vi "Constructor.vi"(8 "error in (no error)":errorcluster, 11 "MallardDuck in":refnum<class "MallardDuck.lvclass">) -> (0 "error out":errorcluster, 3 "MallardDuck out":refnum<class "MallardDuck.lvclass">)   [LabVIEW 2013, in "MallardDuck.lvclass"]
uses:
  MallardDuck.lvclass
  FlyWithWings/FlyWithWings.lvclass
  Quack/Quack.lvclass
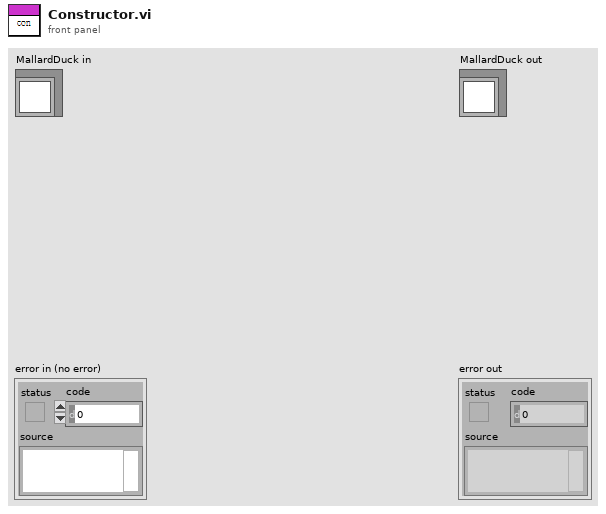
[diagram p1: front panel]
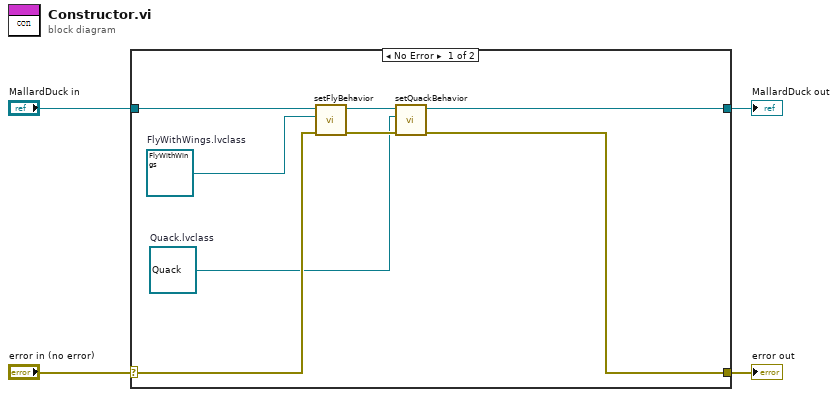
[diagram p0: block diagram]
diagram:
  n1 = case shown="No Error" "error in (no error)" {
    selector: "error in (no error)" -> [w8 w14]
    tunnel: [w7 w14] -> w3
    tunnel: [w10 w13] -> w1
    tunnel: "MallardDuck in" -> [w11 w13]
    frame No Error {
      w5 = refnum<class "Quack.lvclass"> refnum  # Quack.lvclass
      w6 = refnum<class "FlyWithWings.lvclass"> refnum  # FlyWithWings.lvclass
      n2 = call-dynamic "setFlyBehavior.vi"("error in (no error)"=w8, "FlyBehavior.lvclass"=w6, "Duck in"=w11) -> ("error out"=w9:errorcluster, "Duck out"=w12:refnum<class "MallardDuck.lvclass">)  [unwired: 7 in]
      n3 = call-dynamic "setQuackBehavior.vi"("error in (no error)"=w9, "QuackBehavior.lvclass"=w5, "Duck in"=w12) -> ("error out"=w7:errorcluster, "Duck out"=w10:refnum<class "MallardDuck.lvclass">)  [unwired: 7 in]
    }
    frame Error {
    }
  }
  "error out" <- w3
  "MallardDuck out" <- w1
